vi "setCapStyle.vi"(8 "Error In":errorcluster, 10 "capStyle":T1 items=["FlatCap"=0, "SquareCap"=16, "RoundCap"=32, "MPenCapStyle"=48], 11 "QPen In":refnum<class "QPen.lvclass">) -> (0 "Error Out":errorcluster, 3 "QPen Out":refnum<class "QPen.lvclass">)   [LabVIEW 2014, in "QPen.lvclass"]
doc: "LabVIEW-specific documentation is not yet available. See <b>https://doc.qt.io/qt-5/qpen.html#setCapStyle</b>"
uses:
  QPen.lvclass
  LQ Core/Qt/PenCapStyle.ctl
  LQ Core/LQSerialData/LQSerialData.lvclass/LQSerialData.ctl
  LQ Core/LQ Core.lvlib
  LQ Core/LQSerialData/LQSerialData.lvclass
  LQ Core/Qt/Qt.lvlib
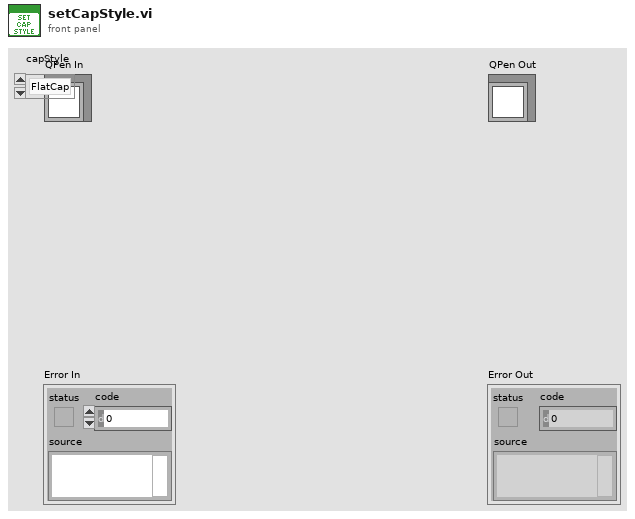
[diagram p1: front panel]
types:
  T1 = typedef "Qt.lvlib/PenCapStyle.ctl" = i32
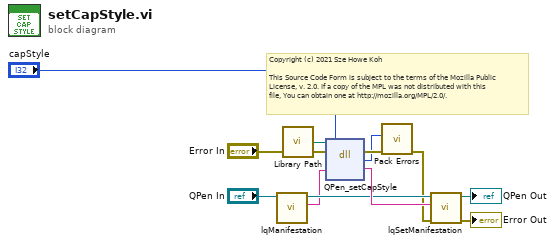
[diagram p0: block diagram]
diagram:
  # "Copyright (c) 2021 Sze Howe Koh\n\nThis Source Code Form is subject to the terms of the Mozilla Public\nLicense, v. 2.0. If a copy of the MPL was not distributed with this\nfile, You can obtain one at http://mozilla.org/MPL/2.0/."
  n1 = call "lqManifestation.vi"("LQSerialData in"="QPen In") -> ("Manifestation"=w7:string, "LQSerialData out"=w8:refnum<class "QPen.lvclass">)  [unwired: 9 in]
  n2 = call "Library Path.vi"() -> ("Library Path"=w6:path)
  n3 = dll-call lib="?" fn="QPen_setCapStyle"(path in=w6, error in="Error In", "_instance"=w7, "capStyle"="capStyle") -> (error out=w5:errorcluster, w4:i32, "_instance"=w10:string)  [unwired: 2 in, 1 out]
  n4 = call "Pack Errors.vi"("Error In"=w5, "Error Code"=w4) -> ("Error Out"=w3:errorcluster)  [unwired: 9 in]
  n5 = call "lqSetManifestation.vi"("Error In"=w3, "Manifestation"=w10, "LQSerialData in"=w8) -> ("Error Out"=→"Error Out":errorcluster, "LQSerialData out"=→"QPen Out":refnum<class "QPen.lvclass">)  [unwired: 7 in]
